vi "Build Google Campaign URL.vi"(4 "Campaign Content":string, 6 "Campaign Term":string, 7 "Campaign Medium":string, 8 "Error In":errorcluster, 9 "Campaign Source":string, 10 "Campaign Name":string, 11 "URL":string) -> (0 "Error Out":errorcluster, 3 "Campaign URL":string)   [LabVIEW 2011, in "LVH-Toolbox.lvlib" / "LVH-SystemTools.lvlib"]
uses:
  LVH-SystemTools.lvlib
  <vilib>/wsapi/NI_WebServices.lvlib
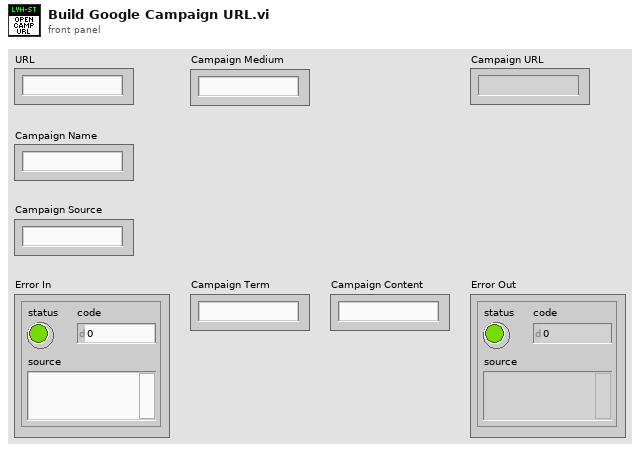
[diagram p1: front panel]
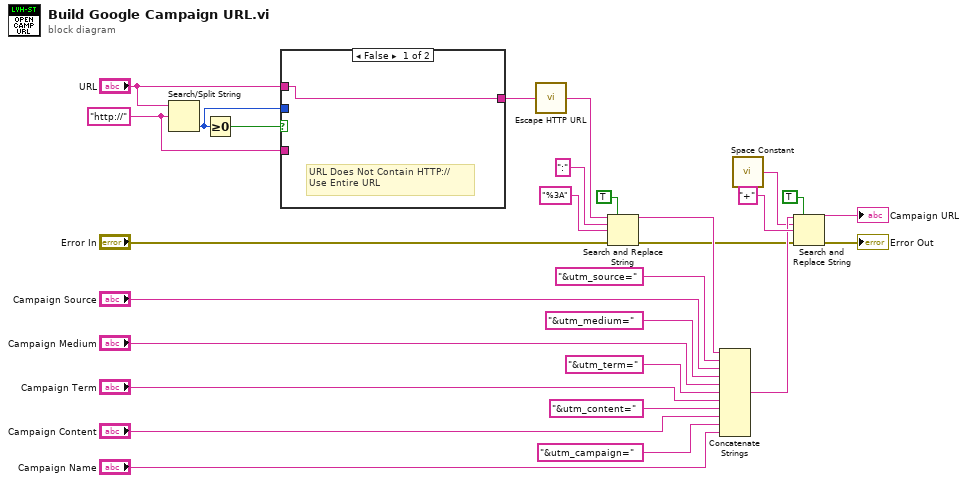
[diagram p0: block diagram]
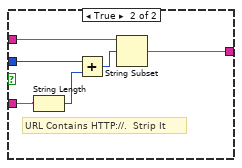
[diagram p2: hidden frame]
diagram:
  w2 = "http://" ("regular expression")
  n1 = Search/Split String(string="URL", search string/char (-)=w2) -> (offset of match=w4:i32)  [unwired: 1 in, 2 out]
  n2 = Greater Or Equal To 0?(x=w4) -> (x >= 0?=w5:bool)
  n3 = case shown="False" w5 {
    tunnel: w4 -> [_ w32]
    tunnel: "URL" -> [w29 w35]
    tunnel: w2 -> [_ w34]
    tunnel: [w29 w30] -> w1
    frame False {
      # "URL Does Not Contain HTTP://\nUse Entire URL"
    }
    frame True {
      # "URL Contains HTTP://.  Strip It"
      n4 = String Length(string=w34) -> (length=w33:i32)
      n5 = Add(x=w32, y=w33) -> (x+y=w31:i32)
      n6 = String Subset(string=w35, offset (0)=w31) -> (substring=w30:string)  [unwired: 1 in]
    }
  }
  n7 = call <vilib>:"Escape HTTP URL.vi"("unescaped string in"=w1) -> ("escaped string out"=w28:string)
  n8 = Search and Replace String(replace all?=TRUE ("replace all? (F)"), input string=w28, search string=":", replace string="%3A" ("replace string (\"\")"), error in="Error In") -> (result string=w23:string, error out=w9:errorcluster)  [unwired: 3 in, 2 out]
  n9 = Concatenate Strings(w23, "&utm_source=" ("string"), "Campaign Source", "&utm_medium=" ("string"), "Campaign Medium", "&utm_term=" ("string"), "Campaign Term", "&utm_content=" ("string"), "Campaign Content", "&utm_campaign=" ("string"), "Campaign Name") -> (w10:string)
  n10 = call <vilib>:"Space Constant.vi"() -> ("String"=w6:string)
  n11 = Search and Replace String(replace all?=TRUE ("replace all? (F)"), input string=w10, search string=w6, replace string="+" ("replace string (\"\")"), error in=w9) -> (result string=→"Campaign URL":string, error out=→"Error Out":errorcluster)  [unwired: 3 in, 2 out]
